vi "ReadFromCSV.vi"(1 "Pages":refnum<vi>[](array[refnum]), 2 "file path (dialog if empty)":path) -> ()   [LabVIEW 2019]
uses:
  <vilib>/Utility/file.llb/Read Delimited Spreadsheet (string).vi
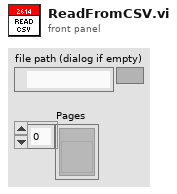
[diagram p1: front panel]
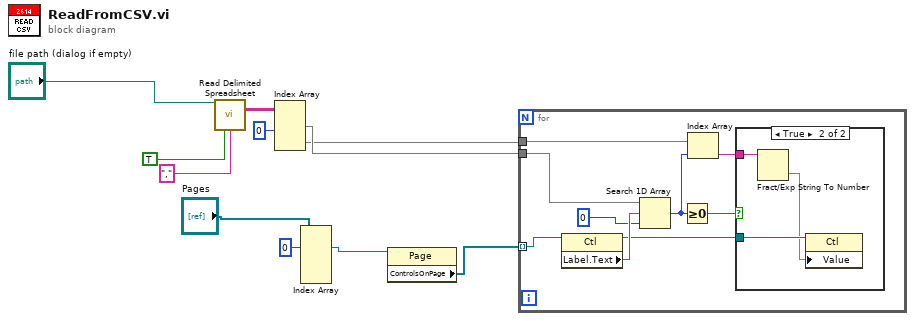
[diagram p0: block diagram]
diagram:
  n1 = call-poly <vilib>:"Read Delimited Spreadsheet.vi"("file path (dialog if empty)"="file path (dialog if empty)", "transpose? (F)"=TRUE, "delimiter (\\t)"="," ("delimiter (\\t)")) -> ("all rows"=w6:string[][])  [unwired: 7 in, 5 out]
  n2 = Index Array(array=w6, index (col) #1=0 ("disabled index (col)")) -> (element #1=w5:string[], element #2=w4:string[])  [unwired: 3 in]
  n3 = Index Array(array="Pages", index #1=0 ("index")) -> (element #1=w3:refnum<vi>)  [unwired: 4 in, 4 out]
  n4 = property class="Page"(reference=w3) -> ("ControlsOnPage"=w1:refnum<vi>[])  [unwired: 1 in, 2 out]
  n5 = for {
    tunnel: w5 -> [w16]
    tunnel: w4 -> [w13]
    tunnel: w1 -> [w12] mode=indexing
    n6 = property class="Ctl"(reference=w12) -> (reference out=w18:refnum<vi>, "Label.Text"=w20:string)  [unwired: 1 in, 1 out]
    n7 = Search 1D Array(1D array=w16, element=w20, start index (0)=0) -> (index of element=w15:i32)
    n8 = Greater Or Equal To 0?(x=w15) -> (x >= 0?=w17:bool)
    n9 = Index Array(array=w13, index=w15) -> (element=w14:string)
    n10 = case shown="True" w17 {
      tunnel: w18 -> [_ w23]
      tunnel: w14 -> [_ w21]
      frame False {
      }
      frame True {
        n11 = Fract/Exp String To Number(string=w21) -> (number=w22:dbl)  [unwired: 3 in, 1 out]
        n12 = property class="Ctl"(reference=w23, "Value"=w22) -> ()  [unwired: 1 in, 2 out]
      }
    }
  }
